vi "Format Date to SQL String.vi"(10 "Month":T1(ring), 11 "YYYY":i32=2008) -> (3 "SQL Date":string)   [LabVIEW 2018]
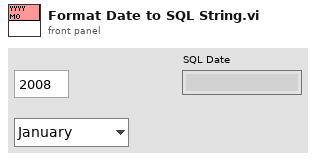
[diagram p1: front panel]
types:
  T1 = enum16{"January", "February", "March", "April", "May", "June", "July", "August", "September", "October", "November", "December"}
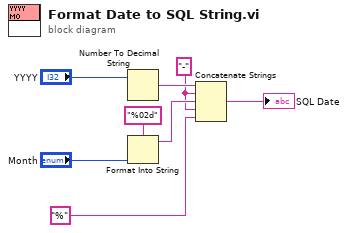
[diagram p0: block diagram]
diagram:
  w3 = "-" ("string")
  n1 = Number To Decimal String(number="YYYY") -> (decimal integer string=w7:string)  [unwired: 1 in]
  n2 = Format Into String(format string="%02d" ("string"), "Month") -> (resulting string=w4:string)  [unwired: 2 in, 1 out]
  n3 = Concatenate Strings(w7, w3, w4, w3, "%" ("string")) -> (→"SQL Date":string)
